vi "DriveDistanceX.vi"(2 "Parameter String":string, 3 "Reinit":bool) -> (0 "Error Out":errorcluster, 1 "Increment":bool)   [LabVIEW 2019]
doc: "The swerve drive base will translate in the field-centric X direction at a speed specified by the joystick command. This is a \"dumb\" algorithm, there is no feedback controller and the direction of translation must be specified manually. Any complex or critical translations should be handled using either the Path Follower or auto-targeting. \n\nParameters:\n1. relative travel distance in the field-centric X direction --> (in) [0,630]\n2. relative translation speed --> [-1,1]"
uses:
  SafeParser_Float.vi
  dscommands.vi
  sensors.vi
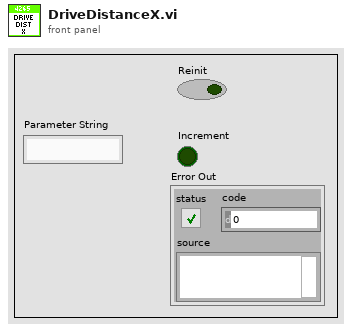
[diagram p1: front panel]
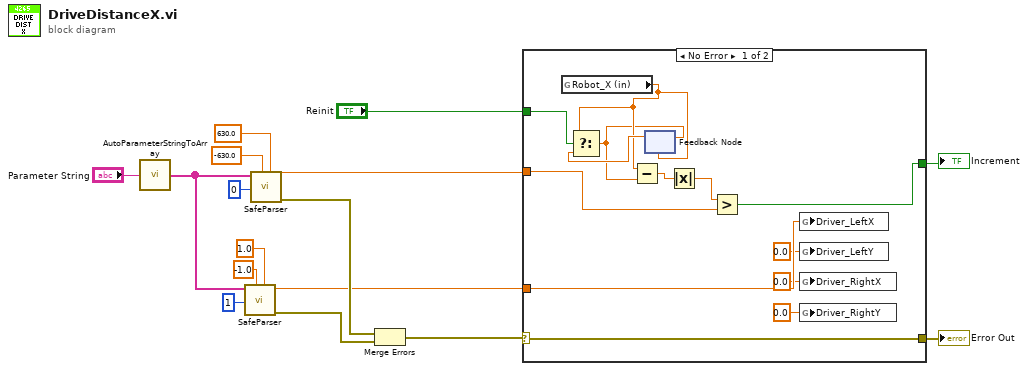
[diagram p0: block diagram]
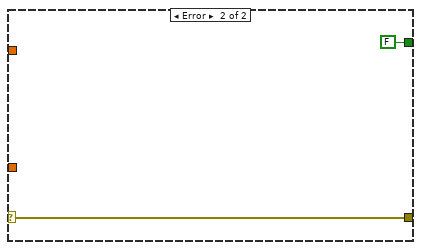
[diagram p2: hidden frame]
diagram:
  n1 = call "AutoParameterStringToArray.vi"("Parameter String"="Parameter String") -> ("Parsed Parameters"=w8:string[])
  n2 = call-poly "SafeParser.vi"("Maximum"=1.0, "Minimum"=-1.0, "Array Index"=1 ("Parameter Index"), "String Array"=w8) -> ("Error Out"=w6:errorcluster, "Typecast  Value"=w3:dbl)  [unwired: 6 in]
  n3 = call-poly "SafeParser.vi"("Maximum"=630.0, "Minimum"=-630.0, "Array Index"=0 ("Parameter Index"), "String Array"=w8) -> ("Error Out"=w5:errorcluster, "Typecast  Value"=w7:dbl)  [unwired: 6 in]
  n4 = Merge Errors(w5, w6) -> (w4:errorcluster)
  n5 = case shown="No Error" w4 {
    selector: w4 -> [w29 w31]
    tunnel: [w25 FALSE] -> w16
    tunnel: "Reinit" -> [w24 _]
    tunnel: [w29 w31] -> w14
    tunnel: w7 -> [w26 _]
    tunnel: w3 -> [w22 _]
    frame No Error {
      n6 = global read "sensors.vi" "Robot_X (in)"() -> (w18:dbl)
      n7 = feedback #1(w18) -> (w23:dbl)
      n8 = Select(t=w18, s=w24, f=w23) -> (s? t:f=w17:dbl)
      n9 = Subtract(x=w18, y=w17) -> (x-y=w28:dbl)
      n10 = feedback-in #1(w17) -> ()
      n11 = Absolute Value(x=w28) -> (abs(x)=w27:dbl)
      n12 = Greater?(x=w27, y=w26) -> (0:w25:bool)
      n13 = global write "dscommands.vi" "Driver_LeftX"(w22) -> ()
      n14 = global write "dscommands.vi" "Driver_LeftY"(0.0 ("Driver_LeftY")) -> ()
      n15 = global write "dscommands.vi" "Driver_RightX"(0.0 ("Driver_RightX")) -> ()
      n16 = global write "dscommands.vi" "Driver_RightY"(0.0 ("Driver_RightY")) -> ()
    }
    frame Error {
    }
  }
  "Increment" <- w16
  "Error Out" <- w14
